vi "window.vi"(8 "error in (no error)":errorcluster caption="错误输入（无错误）", 11 "NormalSetting 输入":refnum<class "NormalSetting.lvclass">) -> (0 "error out":errorcluster caption="错误输出", 3 "NormalSetting 输出":refnum<class "NormalSetting.lvclass">)   [LabVIEW 2015, in "TestLib.lvlib" / "NormalSetting.lvclass"]
uses:
  NormalSetting.lvclass
  NormalSetting.lvclass/NormalSetting.ctl
panel:
  out "路径":path
  in  "字符串":string
  out "布尔":bool
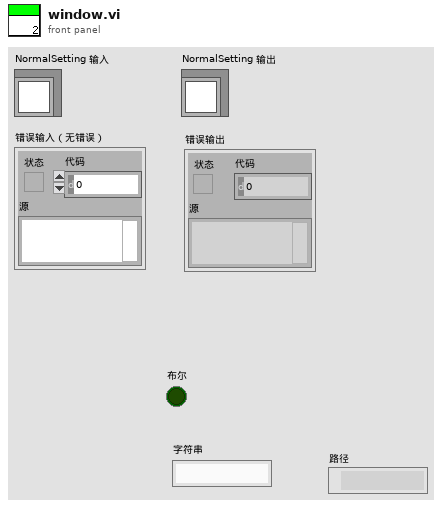
[diagram p1: front panel]
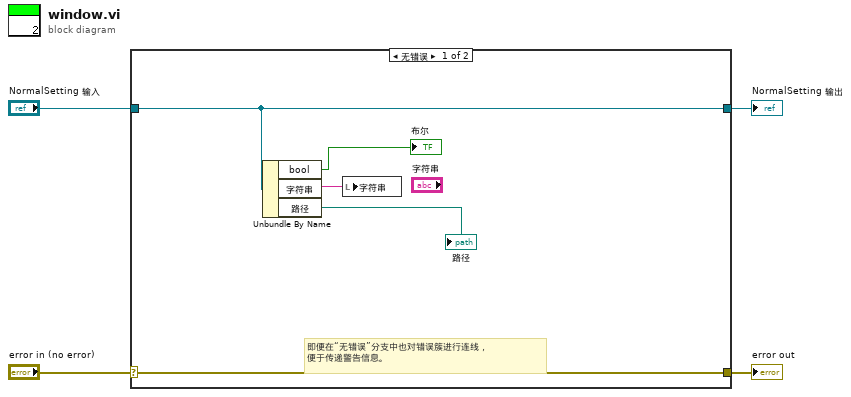
[diagram p0: block diagram]
diagram:
  n1 = case shown="无错误" "error in (no error)" {
    selector: "error in (no error)" -> [w9 w11]
    tunnel: [w9 w11] -> w3
    tunnel: [w8 w10] -> w1
    tunnel: "NormalSetting 输入" -> [w8 w10]
    frame No Error {
      # "即便在“无错误”分支中也对错误簇进行连线，\n便于传递警告信息。"
      n2 = Unbundle By Name(w8) -> ("bool"=→"布尔":bool, "字符串"=w6:string, "路径"=→"路径":path)
      n3 = local write "字符串"(w6) -> ()
    }
    frame Error {
    }
  }
  "error out" <- w3
  "NormalSetting 输出" <- w1
